vi "Simple Temp DataloggerTS.vi"(0 "Thermometer":dbl(slide) scale=0.0..100.0, 3 "datalog path (use dialog)":path) -> ()   [LabVIEW 2011]
doc: "Writes a simulated temperature reading and a timestamp for the reading to a datalog file. Use the Simple Temp Datalog Reader VI in this LLB to read the file."
panel:
  out "Datalog Cluster":T1 {"Temperature" format="%0.2f"}
  # "Press <ctrl-h> for more information."
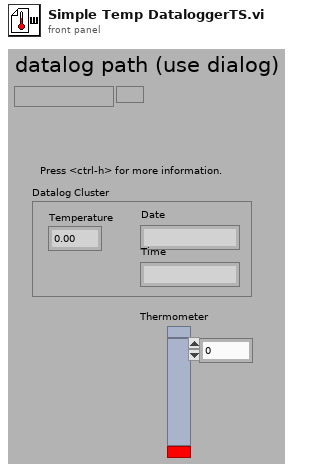
[diagram p1: front panel]
types:
  T1 = cluster{"Temperature":dbl, "Date":string, "Time":string}
  T2 = enum16{"open", "replace", "create", "open or create", "replace or create", "replace or create with confirmation"}
  T3 = cluster{"Thermometer":dbl, "date string":string, "time string":string}
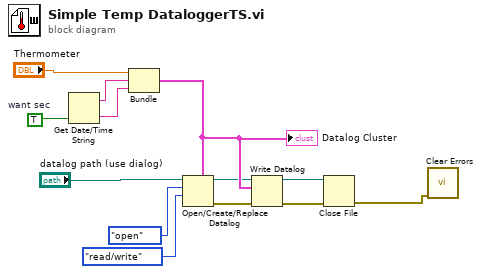
[diagram p0: block diagram]
diagram:
  w11 = TRUE  # want sec
  n1 = Get Date/Time String(want seconds? (F)=w11) -> (date string=w12:string, time string=w13:string)  [unwired: 2 in]
  n2 = Bundle "Bundle"("Thermometer"="Thermometer", "date string"=w12, "time string"=w13) -> (w7:T3)  [unwired: 1 in]
  "Datalog Cluster" <- w7
  n3 = Open/Create/Replace Datalog(5:w7, 9:enum16{"read/write", "read-only", "write-only"}."read/write" ("access (0:read/write)"), 10:T2."open" ("operation (0:open)"), 11:"datalog path (use dialog)") -> (0:w9:errorcluster, 3:w2:refnum<k1>)  [unwired: 2 in, 1 out]
  n4 = Write Datalog(4:w9, 6:w7, 7:w2) -> (0:w8:errorcluster, 3:w10:refnum<k1>)
  n5 = Close File(refnum=w10, error in=w8) -> (error out=w1:errorcluster)  [unwired: 1 out]
  n6 = call <vilib>:"Clear Errors.vi"("error in (no error)"=w1) -> ()  [unwired: 6 in, 1 out]
